vi "Convert Coorninates.vi"(10 "Array":T2(array[cluster])) -> (2 "Array 2":T1[](array[typedef]), 4 "Target Number":i32[](array[numeric]))   [LabVIEW 2023]
uses:
  Target Fields.ctl
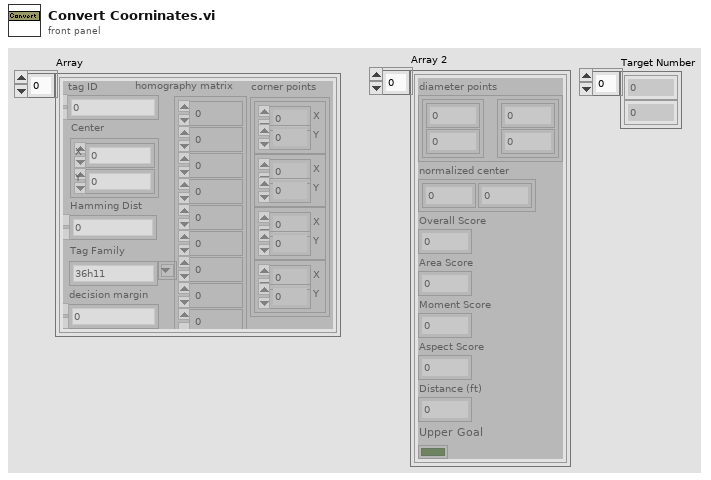
[diagram p1: front panel]
types:
  T1 = typedef "Target Fields.ctl" = cluster{"diameter points":cluster{"first point":cluster{"x":dbl, "y":dbl}, "projected point":cluster{"x":dbl, "y":dbl}}, "normalized center":cluster{"x":dbl, "y":dbl}, "Overall Score":dbl, "Area Score":dbl, "Moment Score":dbl, "Aspect Score":dbl, "Distance (ft)":dbl, "Upper Goal":bool}
  T2 = cluster{"tag ID":i32, "Center":cluster{"X":dbl, "Y":dbl}, "homography matrix":dbl[], "decision margin":dbl, "Hamming Dist":i32, "corner points":cluster{"X":dbl, "Y":dbl}[], "Tag Family":string}[]
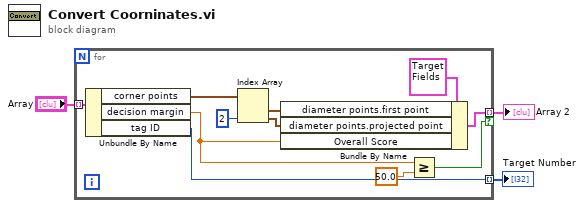
[diagram p0: block diagram]
diagram:
  n1 = for {
    tunnel: [w9] -> w2 mode=indexing if=w5
    tunnel: "Array" -> [w8] mode=indexing
    tunnel: [w4] -> w1 mode=indexing
    n2 = Unbundle By Name(w8) -> ("corner points"=w14:cluster{"X":dbl, "Y":dbl}[], "decision margin"=w7:dbl, "tag ID"=w4:i32)
    n3 = Index Array(array=w14, index #2=2 ("index")) -> (element #1=w12:cluster{"X":dbl, "Y":dbl}, element #2=w11:cluster{"X":dbl, "Y":dbl})  [unwired: 1 in]
    n4 = Bundle By Name(cluster=T1 {"diameter points"={"first point"={"x"=0.0, "y"=0.0}, "projected point"={"x"=0.0, "y"=0.0}}, "normalized center"={"x"=0.0, "y"=0.0}, "Overall Score"=0.0, "Area Score"=0.0, "Moment Score"=0.0, "Aspect Score"=0.0, "Distance (ft)"=0.0, "Upper Goal"=FALSE} ("results"), "diameter points.first point"=w12, "diameter points.projected point"=w11, "Overall Score"=w7) -> (w9:T1)
    n5 = Greater Or Equal?(x=w7, y=50.0) -> (x >= y?=w5:bool)
  }
  "Array 2" <- w2
  "Target Number" <- w1
